vi "Read.vi"(11 "Spawn in":refnum<class "Spawn.lvclass">) -> (2 "Spawn":T1)   [LabVIEW 2025, in "jettl.lvlib" / "Spawn.lvlib" / "Spawn.lvclass"]
uses:
  Spawn.lvclass
  Attributes/Attributes/Attributes.lvclass
  Spawn.ctl
  Spawn.lvlib
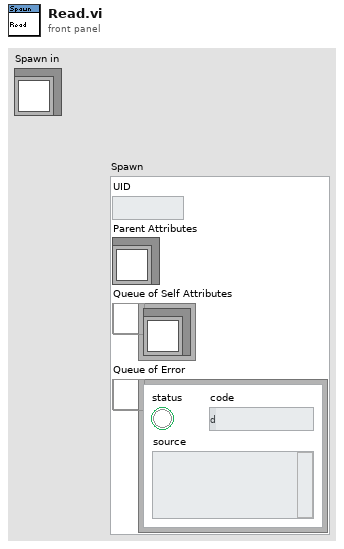
[diagram p1: front panel]
types:
  T1 = typedef "jettl.lvlib/Spawn.lvlib/Spawn.ctl" = cluster{"UID":string, "Parent Attributes":refnum<class "Attributes.lvclass">, "Queue of Self Attributes":refnum<queue>, "Queue of Error":refnum<queue>}
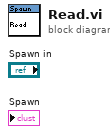
[diagram p0: block diagram]
diagram:
